vi "Get All Dynamic Dispatch Controls.vi"(8 "error in (no error)":errorcluster, 11 "VI in":refnum<vi>) -> (0 "error out":errorcluster, 2 "Dynamic Dispatch Controls":refnum<vi>[](array[refnum]), 3 "reference out":refnum<vi>)   [LabVIEW 2020, in "Responsive Mock Class Generator.lvclass"]
uses:
  Responsive Mock Class Generator.lvclass
  Responsive Mock Class Generator.lvclass/Responsive Mock Class Generator.ctl
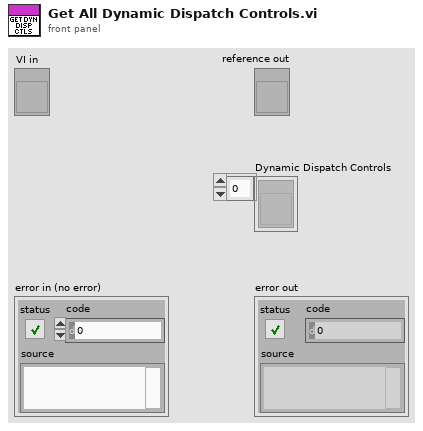
[diagram p1: front panel]
types:
  T1 = enum16{"Invalid Wire Rule", "Required", "Recommended", "Optional", "Dynamic Dispatch"}[]
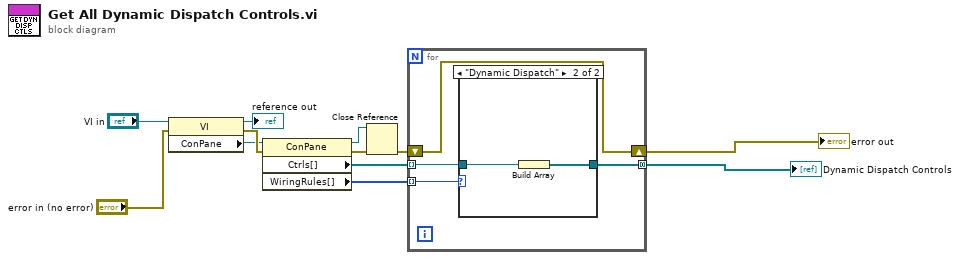
[diagram p0: block diagram]
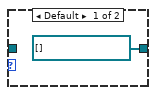
[diagram p2: hidden frame]
diagram:
  n1 = property class="VI"(reference="VI in", error in="error in (no error)") -> (reference out=→"reference out":refnum<vi>, error out=w10:errorcluster, "ConPane"=w5:refnum<vi>)
  n2 = property class="ConPane"(reference=w5, error in=w10) -> (reference out=w1:refnum<vi>, error out=w9:errorcluster, "Ctrls[]"=w6:refnum<vi>[], "WiringRules[]"=w7:T1)
  n3 = Close Reference(reference=w1, error in (no error)=w9) -> (error out=w2:errorcluster)
  n4 = for {
    tunnel: w6 -> [w16] mode=indexing
    tunnel: w7 -> [w15] mode=indexing
    tunnel: [w14] -> w8 mode=concatenating
    shift-right: [w13] -> w12
    shift-left: w2 -> [w13]
    n5 = case shown="\"Dynamic Dispatch\"" w15 {
      tunnel: w16 -> [_ w19]
      tunnel: [refnum<vi>[] [] w18] -> w14
      frame Default {
      }
      frame "Dynamic Dispatch" {
        n6 = Build Array(w19) -> (w18:refnum<vi>[])
      }
    }
  }
  "error out" <- w12
  "Dynamic Dispatch Controls" <- w8
